vi "OK Pressed.vi"(9 "Controls in":refnum<vi>[](array[refnum]), 10 "OK Ref":refnum<vi>) -> ()   [LabVIEW 2020, in "_Shared.lvlib"]
uses:
  _Shared.lvlib
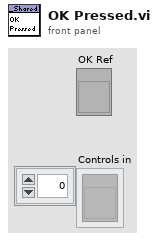
[diagram p1: front panel]
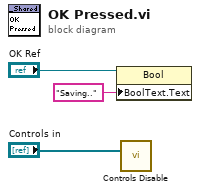
[diagram p0: block diagram]
diagram:
  n1 = property class="Bool"(reference="OK Ref", "BoolText.Text"="Saving.." ("Boolean Text.Text")) -> ()  [unwired: 1 in, 2 out]
  n2 = call "Controls Disable.vi"("Controls in"="Controls in") -> ()  [unwired: 11 in]
